vi "Init Buttons.vi"(8 "error in (no error)":errorcluster, 11 "Refs In":refnum<vi>[](array[refnum])) -> (0 "error out":errorcluster)   [LabVIEW 2013]
doc: "This VI resets all protocol button arrays because it is not possible to change the mechanical action of switches inside an array."
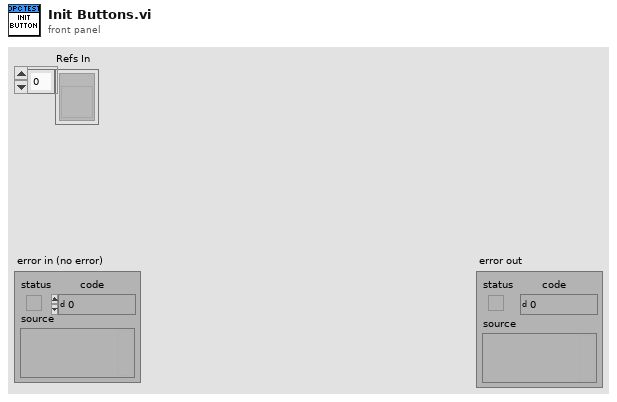
[diagram p1: front panel]
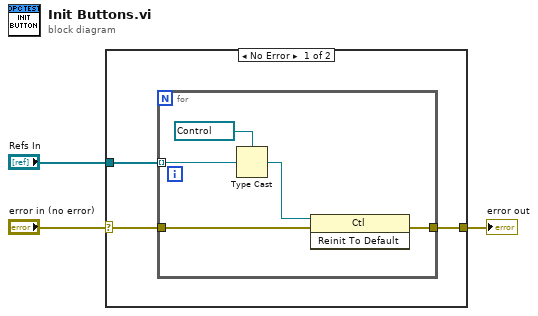
[diagram p0: block diagram]
diagram:
  n1 = case shown="No Error" "error in (no error)" {
    selector: "error in (no error)" -> [w6 w12]
    tunnel: [w5 w12] -> w2
    tunnel: "Refs In" -> [w4 _]
    frame No Error {
      n2 = for {
        tunnel: w4 -> [w10] mode=indexing
        tunnel: w6 -> [w8]
        tunnel: [w7] -> w5
        n3 = Type Cast(type=refnum<vi> refnum ("Ctl Refnum"), x=w10) -> (*(type *) &x=w9:refnum<vi>)
        n4 = invoke class="Ctl" method="Reinit To Default"(reference=w9, error in=w8) -> (error out=w7:errorcluster)  [unwired: 1 in, 2 out]
      }
    }
    frame Error {
    }
  }
  "error out" <- w2
